vi "PH_gentec_Powermeter.ProcPeriodic.vi"(0 "i ref in":refnum<vi>, 3 "ms timeout (100)":i32=100, 5 "error in (no error)":errorcluster) -> (14 "i ref out":refnum<vi>, 17 "timed out":bool, 19 "error out":errorcluster)   [LabVIEW 2014, in "PH_gentec_Powermeter.lvlib"]
doc: "This method serves to periodically do things. In this case, it reads the current value from the powermeter. If the Start Stop - value is true, the statistic data is read out as well. Finally, these data is send to own attributes and the GUI elements."
uses:
  PH_gentec_Powermeter.lvlib
  PH_Basics/PH_Powermeter_BaseClass/PH_Powermeter_BaseClass.lvlib
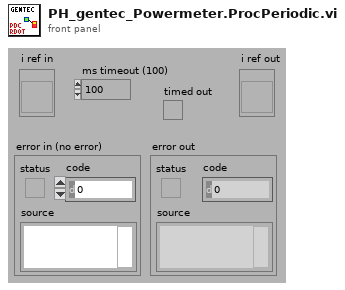
[diagram p1: front panel]
types:
  T1 = typedef "PH_Powermeter_BaseClass.lvlib/PH_Powermeter_BaseClass.State.ctl" = enum32{"off", "operating", "opened", "checked", "connected", "Sets to change", "running"}
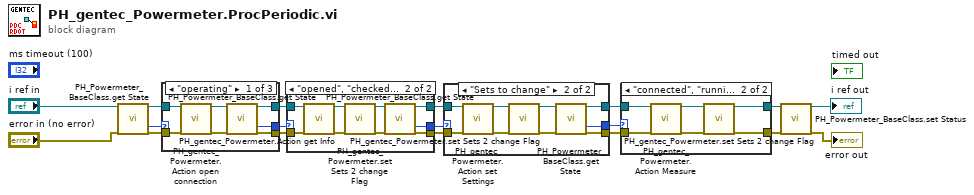
[diagram p0: block diagram]
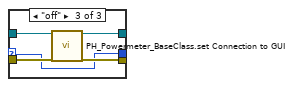
[diagram p6: hidden frame]
diagram:
  n1 = call "PH_Powermeter_BaseClass.get State.vi"("VI in"="i ref in", "error in (no error)"="error in (no error)") -> ("VI out"=w17:refnum<vi>, "State"=w18:T1, "error out"=w16:errorcluster)  [unwired: 14 in, 1 out]
  n2 = case shown="\"operating\"" w18 {
    selector: w18 -> [_ w26 w29]
    tunnel: w17 -> [w24 w28 w33]
    tunnel: w16 -> [w25 w27 w31]
    tunnel: [w21 w27 w30] -> w12
    tunnel: [w22 w28 w32] -> w13
    tunnel: [w19 w26 w29] -> w11
    frame "operating" {
      n3 = call "PH_gentec_Powermeter.Action open connection.vi"("VI in"=w24, "error in (no error)"=w25) -> ("VI out"=w23:refnum<vi>, "error out"=w20:errorcluster)  [unwired: 16 in]
      n4 = call "PH_Powermeter_BaseClass.get State.vi"("VI in"=w23, "error in (no error)"=w20) -> ("VI out"=w22:refnum<vi>, "State"=w19:T1, "error out"=w21:errorcluster)  [unwired: 14 in, 1 out]
    }
    frame Default {
    }
    frame "off" {
      n5 = call "PH_Powermeter_BaseClass.set Connection to GUI.vi"("i ref in"=w33, "error in"=w31) -> ("i ref out"=w32:refnum<vi>, "error out"=w30:errorcluster)  [unwired: 16 in]
    }
  }
  n6 = case shown="\"opened\", \"checked\"" w11 {
    selector: w11 -> [w34 _]
    tunnel: w13 -> [w36 w45]
    tunnel: w12 -> [w35 w44]
    tunnel: [w35 w42] -> w7
    tunnel: [w36 w43] -> w8
    tunnel: [w34 w41] -> w6
    frame Default {
    }
    frame "opened", "checked" {
      n7 = call "PH_gentec_Powermeter.Action get Info.vi"("VI in"=w45, "error in (no error)"=w44) -> ("VI out"=w40:refnum<vi>, "error out"=w38:errorcluster)  [unwired: 16 in]
      n8 = call "PH_gentec_Powermeter.set Sets 2 change Flag.vi"("i ref in"=w40, "error in"=w38) -> ("i ref out"=w39:refnum<vi>, "error out"=w37:errorcluster)  [unwired: 16 in]
      n9 = call "PH_Powermeter_BaseClass.get State.vi"("VI in"=w39, "error in (no error)"=w37) -> ("VI out"=w43:refnum<vi>, "State"=w41:T1, "error out"=w42:errorcluster)  [unwired: 14 in, 1 out]
    }
  }
  n10 = case shown="\"Sets to change\"" w6 {
    selector: w6 -> [w46 _]
    tunnel: w8 -> [w48 w57]
    tunnel: [w48 w56] -> w5
    tunnel: [w47 w55] -> w2
    tunnel: w7 -> [w47 w54]
    tunnel: [w46 w53] -> w1
    frame Default {
    }
    frame "Sets to change" {
      n11 = call "PH_gentec_Powermeter.Action set Settings.vi"("VI in"=w57, "error in (no error)"=w54) -> ("VI out"=w52:refnum<vi>, "error out"=w50:errorcluster)  [unwired: 16 in]
      n12 = call "PH_gentec_Powermeter.set Sets 2 change Flag.vi"("i ref in"=w52, "error in"=w50) -> ("i ref out"=w51:refnum<vi>, "error out"=w49:errorcluster)  [unwired: 16 in]
      n13 = call "PH_Powermeter_BaseClass.get State.vi"("VI in"=w51, "error in (no error)"=w49) -> ("VI out"=w56:refnum<vi>, "State"=w53:T1, "error out"=w55:errorcluster)  [unwired: 14 in, 1 out]
    }
  }
  n14 = case shown="\"connected\", \"running\"" w1 {
    tunnel: [w58 w60] -> w15
    tunnel: [w59 w61] -> w14
    tunnel: w5 -> [w59 w65]
    tunnel: w2 -> [w58 w64]
    frame Default {
    }
    frame "connected", "running" {
      n15 = call "PH_gentec_Powermeter.Action Measure.vi"("VI in"=w65, "error in (no error)"=w64) -> ("VI out"=w63:refnum<vi>, "error out"=w62:errorcluster)  [unwired: 16 in]
      n16 = call "PH_gentec_Powermeter.set Sets 2 change Flag.vi"("i ref in"=w63, "error in"=w62) -> ("i ref out"=w61:refnum<vi>, "error out"=w60:errorcluster)  [unwired: 16 in]
    }
  }
  n17 = call "PH_Powermeter_BaseClass.set Status.vi"("i ref in"=w14, "error in"=w15) -> ("i ref out"=→"i ref out":refnum<vi>, "error out"=→"error out":errorcluster)  [unwired: 16 in]
